vi "Get Addresses.vi"(8 "error in":errorcluster, 11 "AC Comm in":refnum<class "AlicatCommBank.lvclass">=refnum) -> (0 "error out":errorcluster, 2 "Addresses":string[](array[string]), 3 "AC Comm out":refnum<class "AlicatCommBank.lvclass">)   [LabVIEW 2014, in "Alicat.lvlib" / "AlicatCommBank.lvclass"]
uses:
  AlicatCommBank.lvclass
  Alicat.lvclass
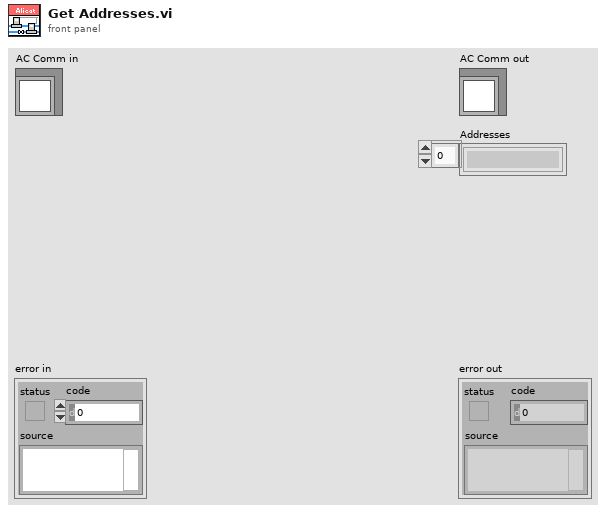
[diagram p1: front panel]
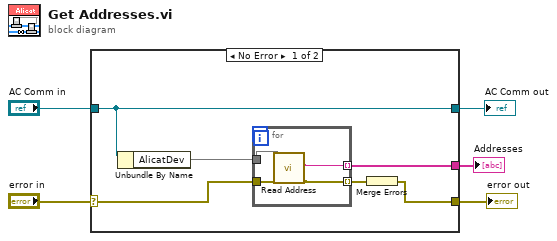
[diagram p0: block diagram]
diagram:
  n1 = case shown="No Error" "error in" {
    selector: "error in" -> [w9 w17]
    tunnel: [w6 w17] -> w1
    tunnel: [w11 w16] -> w3
    tunnel: "AC Comm in" -> [w11 w16]
    tunnel: [w8 _] -> w2
    frame No Error {
      n2 = Unbundle By Name(w11) -> ("AlicatDev"=w10)
      n3 = for {
        tunnel: w10 -> [w15]
        tunnel: w9 -> [w13]
        tunnel: [w12] -> w7 mode=indexing
        tunnel: [w14] -> w8 mode=indexing
        n4 = call "Read Address.vi"("error in"=w13, "Alicat in"=w15) -> ("error out"=w12:errorcluster, "Address"=w14:string)  [unwired: 7 in, 1 out]
      }
      n5 = Merge Errors(w7) -> (w6:errorcluster)
    }
    frame Error {
    }
  }
  "error out" <- w1
  "AC Comm out" <- w3
  "Addresses" <- w2
